vi "Drive Straight (Distance)(SubVI).vi"(6 "Slow Down time":u32, 9 "AutoY":dbl, 10 "Distance":dbl, 11 "DriveMotorRefNum":string="RobotDrive") -> (3 "String":string)   [LabVIEW 2017]
uses:
  <vilib>/Rock Robotics/WPI/SafetyOutput/WPI_SafetyOutputConfigMenu.ctl
  Robot Global Data.vi
  <vilib>/Rock Robotics/WPI/Utilities/WPI_GetSetVariantRefNum.vi
  <vilib>/Rock Robotics/WPI/RobotDrive/WPI_RobotDriveArcadeDrive_Standard(NoSaturation).vi
  <vilib>/Rock Robotics/WPI/RobotDrive/WPI_RobotDriveSafetyCheck.vi
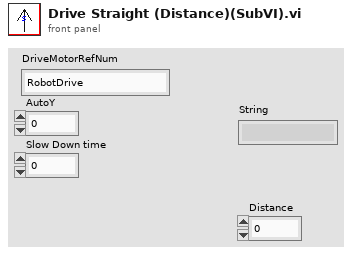
[diagram p1: front panel]
types:
  T1 = typedef "WPI_SafetyOutputConfigMenu.ctl" = enum16{"Enable", "Disable"}
  T2 = typedef "WPI_RobotDriveDevRef.ctl" = cluster{"DevStatus":errorcluster, "Motors[]":T3[], "Square Inputs":bool, "Max Output":dbl}
  T3 = typedef "WPI_MotorControlDeviceRef.ctl" = cluster{"DeviceStatus":errorcluster, "Type":T4, "PWM":cluster{"PWM Channel":T5, "DeadBand":T6}, "CAN":cluster{"Device Number":u8, "SetOutput VI Ref":variant, "GetOutput VI Ref":variant, "Enable VI Ref":variant, "Disable VI Ref":variant, "Data":variant}, "Invert":bool, "DIO PWM":cluster{"PWM \"Enable\" Channel":T5, "DIOChannel":T7, "PWM Rate":dbl}}
  T4 = typedef "WPI_MotorControlType.ctl" = enum16{"PWM", "CAN", "DIO PWM"}
  T5 = typedef "FPGA_DIOPWMChannel.ctl" = enum8{"PWM 0", "PWM 1", "PWM 2", "PWM 3", "PWM 4", "PWM 5", "PWM 6", "PWM 7", "PWM 8", "PWM 9", "PWM MXP 0", "PWM MXP 1", "PWM MXP 2", "PWM MXP 3", "PWM MXP 4", "PWM MXP 5", "PWM MXP 6", "PWM MXP 7", "PWM MXP 8", "PWM MXP 9", "Invalid"}
  T6 = typedef "WPI_PWMDeadband.ctl" = cluster{"Name":string, "maxPositivePwm":i32, "minPositivePwm":i32, "centerPwm":i32, "maxNegativePwm":i32, "minNegativePwm":i32, "angularRange":u16}
  T7 = typedef "FPGA_DIOChannel.ctl" = enum8{"DIO 0", "DIO 1", "DIO 2", "DIO 3", "DIO 4", "DIO 5", "DIO 6", "DIO 7", "DIO 8", "DIO 9", "DIO MXP 0", "DIO MXP 1", "DIO MXP 2", "DIO MXP 3", "DIO MXP 4", "DIO MXP 5", "DIO MXP 6", "DIO MXP 7", "DIO MXP 8", "DIO MXP 9", "DIO MXP 10", "DIO MXP 11", "DIO MXP 12", "DIO MXP 13", "DIO MXP 14", "DIO MXP 15", "SPI Port CS1", "SPI Port CS2", "SPI Port CS3", "SPI Port MISO", "SPI Port MOSI", "Invalid"}
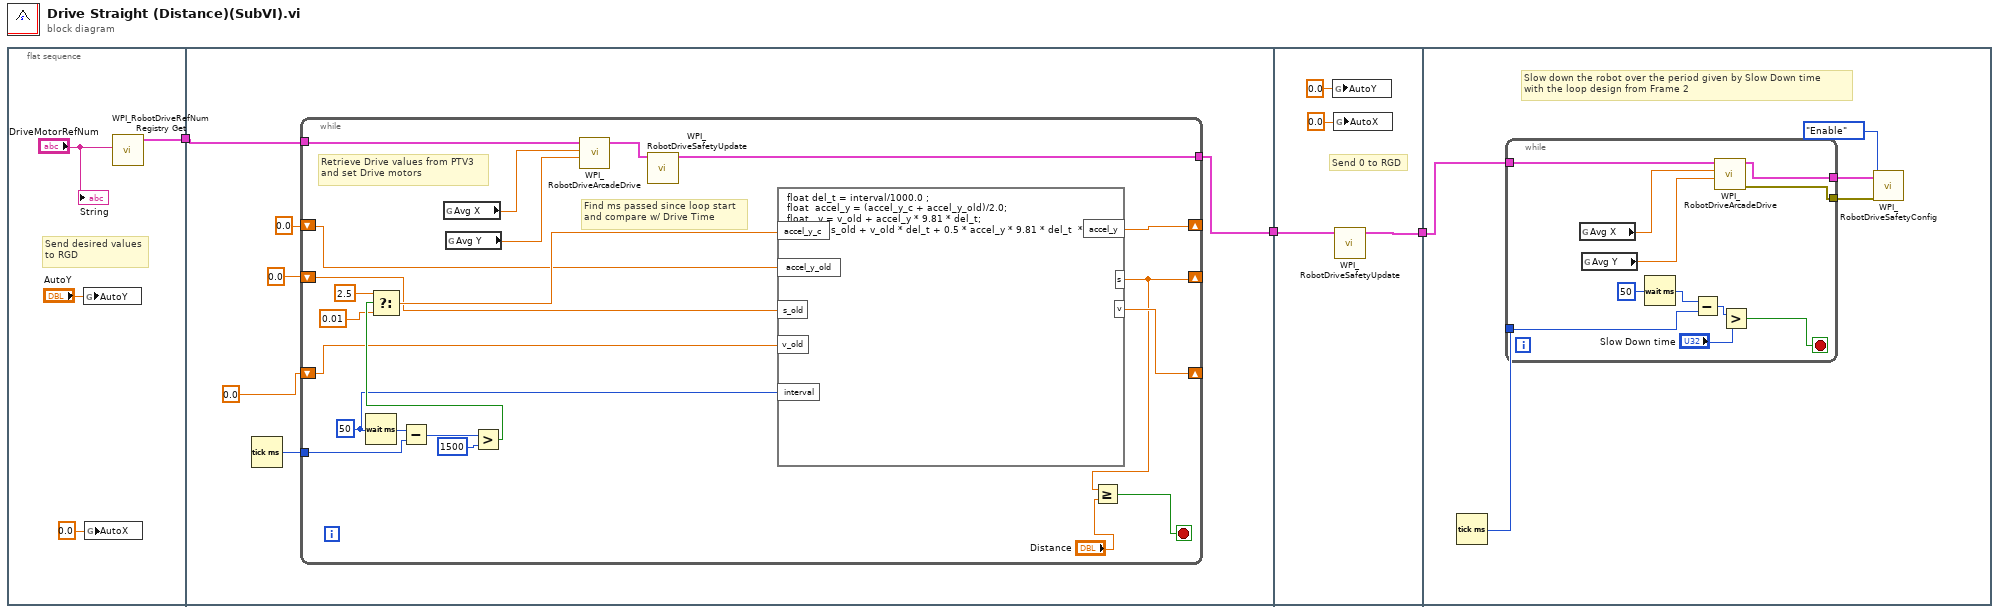
[diagram p0: block diagram]
diagram:
  n1 = flat-sequence {
    tunnel: [w7] -> w3
    tunnel: w3 -> [w12]
    tunnel: [w11] -> w2
    tunnel: [w38] -> w1
    tunnel: w2 -> [w39]
    tunnel: w1 -> [w43]
    frame #0 {
      # "Send desired values\nto RGD"
      n2 = global write "Robot Global Data.vi" "AutoY"("AutoY") -> ()
      n3 = global write "Robot Global Data.vi" "AutoX"(0.0 ("AutoX")) -> ()
      n4 = call <vilib>:"WPI_RobotDriveRefNum Registry Get.vi"("refnum name"="DriveMotorRefNum") -> ("RobotDriveDevRef"=w7:T2)  [unwired: 9 in, 1 out]
      "String" <- "DriveMotorRefNum"
    }
    frame #1 {
      n5 = Tick Count (ms)() -> (millisecond timer value=w13:u32)
      n6 = while {
        tunnel: w12 -> [w33]
        tunnel: [w30] -> w11
        tunnel: w13 -> [w32]
        shift-right: [w23] -> _
        shift-left: 0.0 -> [w22]
        shift-right: [w18] -> _
        shift-left: 0.0 -> [w21]
        shift-right: [w20] -> _
        shift-left: 0.0 -> [w19]
        stop <- w16 stop-if-true
        w24 = u32 50 ("milliseconds to wait")
        # "Retrieve Drive values from PTV3\nand set Drive motors"
        # "Find ms passed since loop start\nand compare w/ Drive Time"
        n7 = Wait (ms)(milliseconds to wait=w24) -> (millisecond timer value=w14:u32)
        n8 = Subtract(x=w14, y=w32) -> (x-y=w15:u32)
        n9 = global read "Robot Global Data.vi" "Avg X"() -> (w35:dbl)
        n10 = global read "Robot Global Data.vi" "Avg Y"() -> (w34:dbl)
        n11 = Greater?(x=w15, y=u32 1500) -> (0:w28:bool)
        n12 = Select(t=2.5, s=w28, f=0.01) -> (s? t:f=w25:dbl)
        n13 = call-poly <vilib>:"WPI_RobotDriveArcadeDrive.vi"("Y axis value"=w34, "X axis value"=w35, "RobotDriveDevRef"=w33) -> ("RobotDriveDevRef"=w31:T2)  [unwired: 6 in, 2 out]
        n14 = call <vilib>:"WPI_RobotDriveSafetyUpdate.vi"("RobotDriveDevRef"=w31) -> ("RobotDriveDevRef"=w30:T2)  [unwired: 1 in, 9 out]
        n15 = formula code="float del_t = interval/1000.0 ;\nfloat  accel_y = (accel_y_c + accel_y_old)/2.0;\nfloat   v = v_old + accel_y * 9.81 * del_t;\nfloat s = s_old + v_old * del_t + 0.5 * accel_y * 9.81 * del_t  * del_t;"("accel_y_c"=w25, "accel_y_old"=w22, "s_old"=w21, "v_old"=w19, "interval"=w24) -> ("accel_y"=w23:dbl, "s"=w18:dbl, "v"=w20:dbl)
        n16 = Greater Or Equal?(x=w18, y="Distance") -> (x >= y?=w16:bool)
      }
    }
    frame #2 {
      # "Send 0 to RGD"
      n17 = global write "Robot Global Data.vi" "AutoY"(0.0 ("AutoY")) -> ()
      n18 = global write "Robot Global Data.vi" "AutoX"(0.0 ("AutoX")) -> ()
      n19 = call <vilib>:"WPI_RobotDriveSafetyUpdate.vi"("RobotDriveDevRef"=w39) -> ("RobotDriveDevRef"=w38:T2)  [unwired: 1 in, 9 out]
    }
    frame #3 {
      # "Slow down the robot over the period given by Slow Down time\nwith the loop design from Frame 2"
      n20 = Tick Count (ms)() -> (millisecond timer value=w44:u32)
      n21 = while {
        tunnel: w43 -> [w53]
        tunnel: [w50] -> w42
        tunnel: w44 -> [w49]
        tunnel: [w47] -> w41
        stop <- w51 stop-if-true
        n22 = global read "Robot Global Data.vi" "Avg X"() -> (w55:dbl)
        n23 = global read "Robot Global Data.vi" "Avg Y"() -> (w54:dbl)
        n24 = Wait (ms)(milliseconds to wait=u32 50) -> (millisecond timer value=w48:u32)
        n25 = Subtract(x=w48, y=w49) -> (x-y=w46:u32)
        n26 = call-poly <vilib>:"WPI_RobotDriveArcadeDrive.vi"("Y axis value"=w54, "X axis value"=w55, "RobotDriveDevRef"=w53) -> ("error out"=w47:errorcluster, "RobotDriveDevRef"=w50:T2)  [unwired: 6 in, 1 out]
        n27 = Greater?(x=w46, y="Slow Down time") -> (0:w51:bool)
      }
      n28 = call <vilib>:"WPI_RobotDriveSafetyConfig.vi"("error in (no error)"=w41, "mode"=WPI_SafetyOutputConfigMenu."Enable", "RobotDriveDevRef"=w42) -> ()  [unwired: 7 in, 2 out]
    }
  }
